vi "TenGbE_FPGA.vi"() -> ()   [LabVIEW 2017, in "My Network FPGA v1.lvlib"]
uses:
  Example SubVIs/My Network FPGA v1.lvlib
  <instrlib>/_niInstr/Streaming/v1/Common/Stream State.ctl
  <vilib>/Platform/TimedLoop/XDataNode/timing_clust.ctl
  <vilib>/Platform/TimedLoop/XDataNode/nitl_modes.ctl
  <vilib>/Platform/TimedLoop/XDataNode/wakeup.ctl
  <instrlib>/_niInstr/Network/Ethernet/MAC/CLIP/v1/Resources.ctl
  Example SubVIs/TX Controls.ctl
  <instrlib>/_niInstr/Network/Ethernet/MAC/CLIP/v1/niInstr Ethernet MAC - CLIP v1.lvclass
  C:/Program Files (x86)/National Instruments/LabVIEW 2017/instr.lib/_niInstr/Network/Ethernet/MAC/API/v1/FPGA/niInstr Ethernet MAC v1.lvclass
  <instrlib>/_niInstr/Network/API/v1/FPGA/Address Space/niInstr Network API FPGA Address Space v1.lvclass
  C:/Program Files (x86)/National Instruments/LabVIEW 2017/instr.lib/_niInstr/Instruction Framework/v1/FPGA/Interfaces/Address Space Collection/Address Space Collection.lvclass
  <instrlib>/_niInstr/FIFO Register Bus/v1/FPGA/niInstr FIFO Register Bus v1 FPGA.lvclass
  C:/Program Files (x86)/National Instruments/LabVIEW 2017/instr.lib/_niInstr/Instruction Framework/v1/FPGA/Interfaces/Instruction Producer/Instruction Producer.lvclass
  <vilib>/rvi/Emulation/niFpgaSctlEmulationGetInTimedLoop.vi
  <vilib>/rvi/Emulation/niFpgaEmulationReportErrorSimple.vi
  <vilib>/rvi/Emulation/niFpgaGetClockAttributes.vi
  <vilib>/rvi/Emulation/niFpgaCriticalErrorInLSC.vi
  <vilib>/rvi/Emulation/niFpgaProcessEmulError.vi
  <vilib>/rvi/eio/common/nirviEmuTemplateMethod_errors.vi
  <vilib>/Platform/TimedLoop/XDataNode/XDataNode.xnode
  <vilib>/eio/EIONode/EIONode.xnode
  <vilib>/Platform/TimedLoop/XDataNode/XDNodeRunTimeDep.lvlib
  <instrlib>/_niInstr/Instruction Framework/v1/FPGA/Top Level Bus/Register Configuration/Register Configuration.lvclass
  <instrlib>/_niInstr/Network/API/v1/FPGA/niInstr Network API FPGA v1.lvclass
  <instrlib>/_niInstr/Streaming/v1/Common/niInstr Streaming v1 Common.lvlib
panel:
  out "d_microblaze\\AXI_STR_RXD_1_tready":bool
  out "d_microblaze\\AXI_STR_RXD_tready":bool
  out "d_microblaze\\AXI_STR_TXD_1_tdata":fxp<+,32,32>
  out "d_microblaze\\AXI_STR_TXD_1_tlast":bool
  out "d_microblaze\\AXI_STR_TXD_1_tvalid":bool
  out "d_microblaze\\AXI_STR_TXD_tdata":fxp<+,32,32>
  out "d_microblaze\\AXI_STR_TXD_tlast":bool
  out "d_microblaze\\AXI_STR_TXD_tvalid":bool
  out "d_microblaze\\gpio1_out_tri_o":fxp<+,32,32>
  out "d_microblaze\\gpio2_out_tri_o":fxp<+,32,32>
  in  "Tab Control":T1(tab)
  in  "UDP Source Port 0":u16=43981
  in  "UDP Destination Port 0":u16=61185
  in  "preferred datagram size 0":u16=1472
  in  "Port 0 RX/TX":enum32{"RX", "TX"}(tab)
  in  "Port 0 RAW Mode":bool
  in  "Port 0 RX Clear Counts":bool
  out "Port 0 RX Good Frames Count":u32
  out "Port 0 RX Error Frames Count":u32
  out "Port 0 RX Received Columns Count":u32
  out "Port 0 RX Dropped Columns Count":u32
  out "Port 0 RX Data":u64 format="%.0x"
  in  "stream.num samples 0":u64
  in  "stream.request state 0":T2
  out "stream.metadata 0":u64
  out "stream.samples transferred 0":u64
  out "stream.state 0":T2
  in  "UDP Source Port 1":u16=43981
  in  "UDP Destination Port 1":u16=61185
  in  "preferred datagram size 1":u16=1472
  in  "Port 1 RX/TX":enum32{"RX", "TX"}(tab)
  in  "Port 1 RAW Mode":bool
  in  "Port 1 RX Clear Counts":bool
  out "Port 1 RX Dropped Columns Count":u32
  out "Port 1 RX Received Columns Count":u32
  out "Port 1 RX Error Frames Count":u32
  out "Port 1 RX Good Frames Count":u32
  out "Port 1 RX Data":u64 format="%.0x"
  in  "stream.request state 1":T2 caption="stream.request state 0"
  in  "stream.num samples 1":u64 caption="stream.num samples 0"
  out "stream.state 1":T2 caption="stream.state 0"
  out "stream.samples transferred 1":u64 caption="stream.samples transferred 0"
  out "stream.metadata 1":u64 caption="stream.metadata 0"
  in  "Use Pattern Gen":bool
  in  "max frame payload":u16=1472
  in  "minimum packet interval":u32=1
  out "mgtrefclks_locked":bool
  out "mgtrefclks_valid":bool
  out "posc_complete":bool
  out "aBlockLockPort0":bool
  out "aBlockLockPort1":bool
  out "sPort0_Power_Good":bool
  out "sPort1_Power_Good":bool
  out "signal_detect_Port0":bool
  out "signal_detect_Port1":bool
  in  "fifo reg bus ctrl 0":u32
  out "fifo reg bus status 0":u32
  out "fifo reg bus data 0":u64
  # "License Note\n\nThis example makes use of code under the LGPLv2 license in the Socketed CLIP to support 10 Gigabit Ethernet.  You may find the source and build instructions for this component in the CLIP directory."
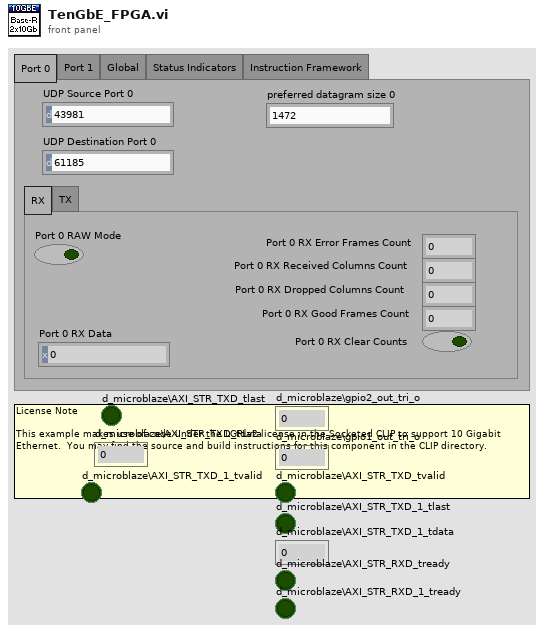
[diagram p1: front panel]
types:
  T1 = enum32{"Port 0", "Port 1", "Global", "Status Indicators", "Instruction Framework"}
  T2 = typedef "niInstr Streaming v1 Common.lvlib/Stream State.ctl" = enum8{"Idle", "Finite Transfer", "Continuous", "Done", "Error", "Not Ready", "Cancel"}
  T3 = typedef "niInstr Ethernet MAC - CLIP v1.lvclass/Resources.ctl" = cluster{"RX":cluster{"TData":refnum<k21>, "TValid":refnum<k21>, "TKeep":refnum<k21>, "TLast":refnum<k21>, "TUser":refnum<k21>}, "TX":cluster{"TData":refnum<k21>, "TValid":refnum<k21>, "TKeep":refnum<k21>, "TLast":refnum<k21>, "TReady":refnum<k21>}, "Pause resources":cluster{"cPauseValuePort":refnum<k21>, "cPauseReqPort":refnum<k21>}, "MAC Clock":refnum<k21>}
  T4 = typedef "XDNodeRunTimeDep.lvlib/timing_clust.ctl" = cluster{"Expected End [f-1]":u64, "Actual End [f-1]":u64, "Finished Late? [f-1]":bool, "Expected End [i-1]":u64, "Actual End [i-1]":u64, "Finished Late? [i-1]":bool, "Expected Start [i]":u64, "Actual Start [i]":u64, "Expected Start [f]":u64, "Actual Start [f]":u64, "Source Name":string, "Structure Name":string, "Period":i64, "Deadline":i64, "Offset":i64, "Start":i64, "Priority":i32, "Timeout":i32, "Mode":T5, "Wakeup Reason":T6, "Error":errorcluster, "Source Type":string, "Secondary Source Type":string, "Global End Time":u64, "Global Start Time":u64, "Frame Duration":u64, "Iteration Duration":u64, "Assigned CPU":i32, "I/O Scan Engine Mode":u32}
  T5 = typedef "XDNodeRunTimeDep.lvlib/nitl_modes.ctl" = enum32{"No Change", "Process missed periods, maintain original phase", "Discard missed periods, maintain original phase", "Process missed periods, ignore original phase", "Discard missed periods, ignore original phase"}
  T6 = typedef "XDNodeRunTimeDep.lvlib/wakeup.ctl" = enum32{"Normal", "Aborted", "Asynchronous wakeup", "Timing source error", "Timed loop error", "Timeout"}
  T7 = typedef "My Network FPGA v1.lvlib/TX Controls.ctl" = cluster{"UDP Source Port":u16, "UDP Destination Port":u16, "preferred datagram size":u16, "Use Pattern Gen":bool, "max frame payload":u16, "minimum packet interval":u32, "stream.num samples 0":u64, "stream.request state 0":T2}
  T8 = cluster{"Port RX Good Frames Count":u32, "Port RX Received Columns Count":u32, "Port RX Dropped Columns Count":u32, "Port RX Error Frames Count":u32, "Port RX Data":u64}
  T9 = typedef "My Network FPGA v1.lvlib/TX Indicators.ctl" = cluster{"stream.state 0":T2, "stream.metadata 0":u64, "stream.samples transferred 0":u64}
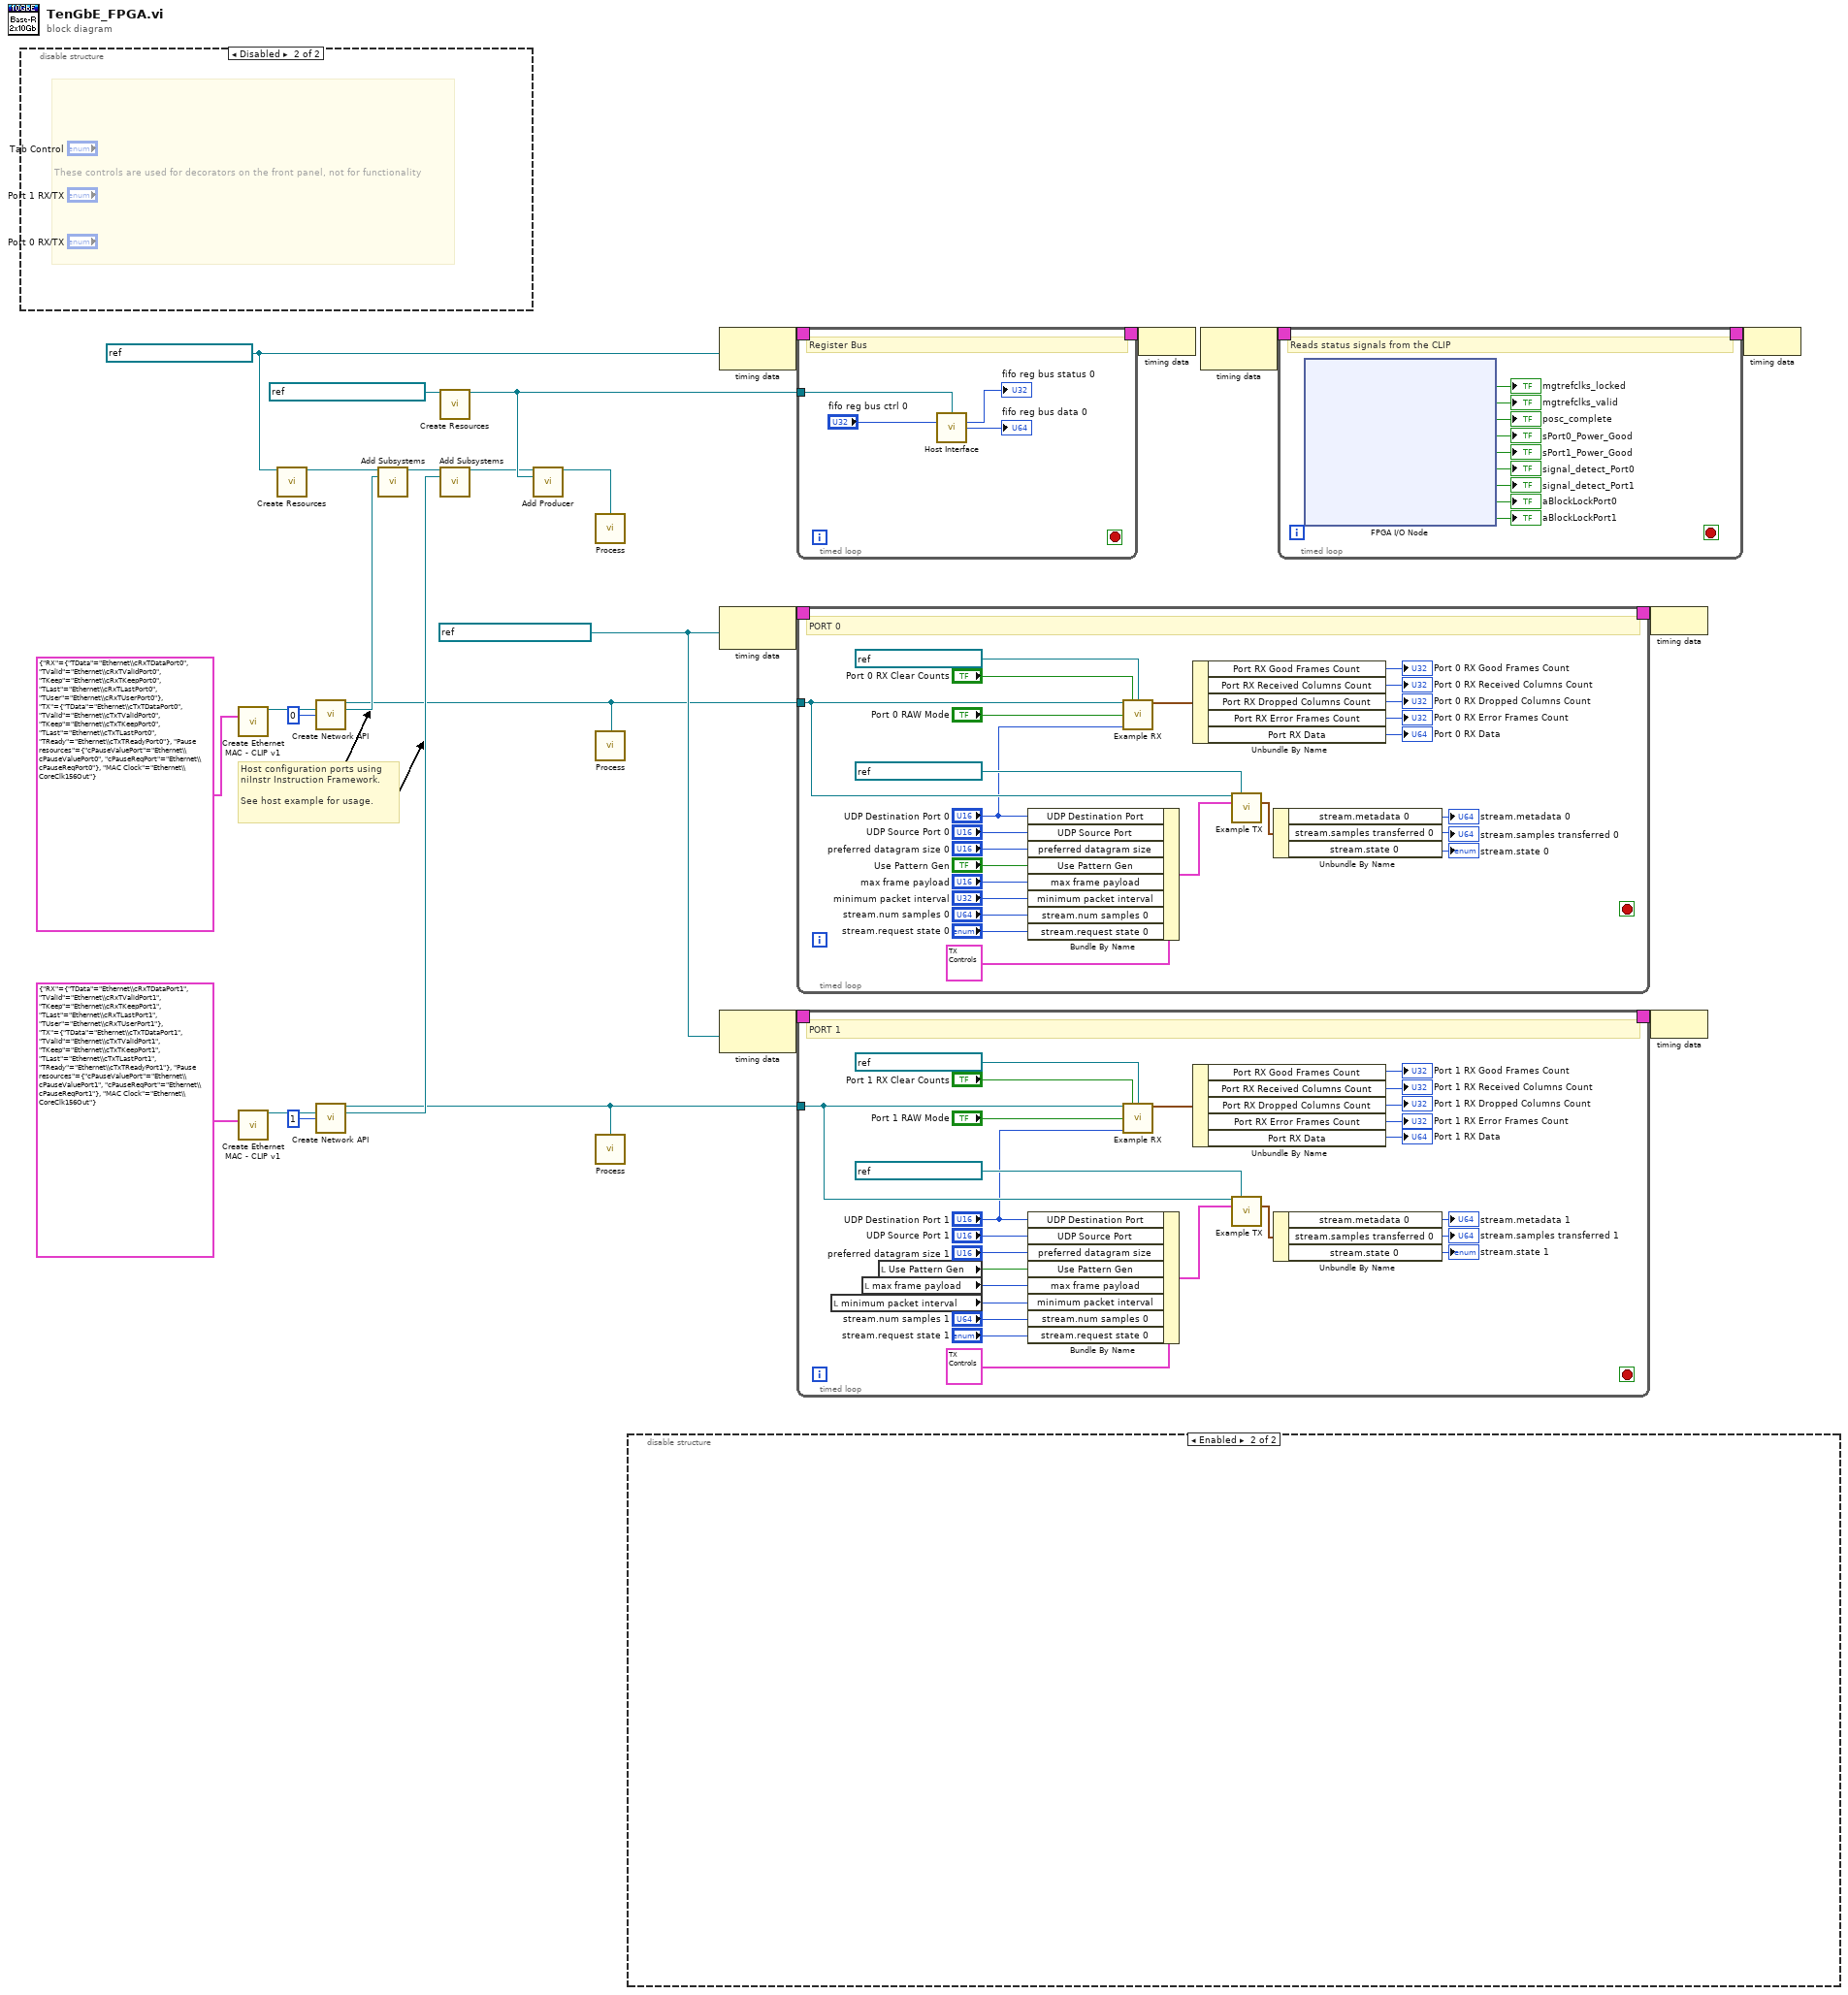
[diagram p0: block diagram]
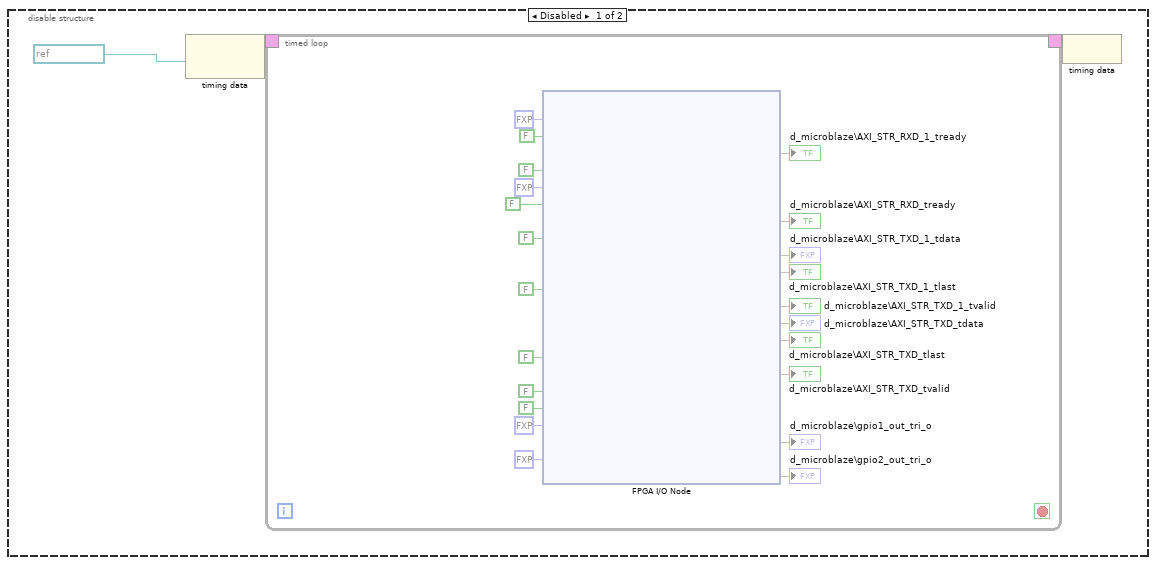
[diagram p2: hidden frame]
diagram:
  w5 = refnum<k21> "Ethernet\\CoreClk156Out" ("Source Name")
  w21 = refnum<k21> "40 MHz Onboard Clock" ("Source Name")
  # "Host configuration ports using\nniInstr Instruction Framework.\n\nSee host example for usage."
  n1 = disable-structure shown="Disabled" {
    frame Enabled {
    }
    frame Disabled {
      # "These controls are used for decorators on the front panel, not for functionality"
    }
  }
  n2 = call <instrlib>:"Create Ethernet MAC - CLIP v1.vi"("Ethernet AXI4-S Resources"=T3 {"RX"={"TData"="Ethernet\\cRxTDataPort0", "TValid"="Ethernet\\cRxTValidPort0", "TKeep"="Ethernet\\cRxTKeepPort0", "TLast"="Ethernet\\cRxTLastPort0", "TUser"="Ethernet\\cRxTUserPort0"}, "TX"={"TData"="Ethernet\\cTxTDataPort0", "TValid"="Ethernet\\cTxTValidPort0", "TKeep"="Ethernet\\cTxTKeepPort0", "TLast"="Ethernet\\cTxTLastPort0", "TReady"="Ethernet\\cTxTReadyPort0"}, "Pause resources"={"cPauseValuePort"="Ethernet\\cPauseValuePort0", "cPauseReqPort"="Ethernet\\cPauseReqPort0"}, "MAC Clock"="Ethernet\\CoreClk156Out"}) -> ("niInstr Ethernet MAC - CLIP v1.lvclass out"=w16:refnum<class "niInstr Ethernet MAC - CLIP v1.lvclass">)  [unwired: 14 in]
  n3 = call <instrlib>:"Create Ethernet MAC - CLIP v1.vi"("Ethernet AXI4-S Resources"=T3 {"RX"={"TData"="Ethernet\\cRxTDataPort1", "TValid"="Ethernet\\cRxTValidPort1", "TKeep"="Ethernet\\cRxTKeepPort1", "TLast"="Ethernet\\cRxTLastPort1", "TUser"="Ethernet\\cRxTUserPort1"}, "TX"={"TData"="Ethernet\\cTxTDataPort1", "TValid"="Ethernet\\cTxTValidPort1", "TKeep"="Ethernet\\cTxTKeepPort1", "TLast"="Ethernet\\cTxTLastPort1", "TReady"="Ethernet\\cTxTReadyPort1"}, "Pause resources"={"cPauseValuePort"="Ethernet\\cPauseValuePort1", "cPauseReqPort"="Ethernet\\cPauseReqPort1"}, "MAC Clock"="Ethernet\\CoreClk156Out"}) -> ("niInstr Ethernet MAC - CLIP v1.lvclass out"=w13:refnum<class "niInstr Ethernet MAC - CLIP v1.lvclass">)  [unwired: 14 in]
  n4 = call <instrlib>:"Create Resources.vi"("register clock"=w21) -> ("register configuration"=w15:refnum<class "Register Configuration.lvclass">)  [unwired: 14 in]
  n5 = call <instrlib>:"Create Network API.vi"("niInstr Ethernet MAC v1.lvclass"=w16, "instance"=u8 0 ("Instance")) -> ("niInstr Network API FPGA v1.lvclass"=w1:refnum<class "niInstr Network API FPGA v1.lvclass">, "Address Space Collection"=w14:refnum<class "niInstr Network API FPGA Address Space v1.lvclass">)  [unwired: 12 in]
  n6 = call <instrlib>:"Create Network API.vi"("niInstr Ethernet MAC v1.lvclass"=w13, "instance"=u8 1 ("Instance")) -> ("niInstr Network API FPGA v1.lvclass"=w4:refnum<class "niInstr Network API FPGA v1.lvclass">, "Address Space Collection"=w11:refnum<class "niInstr Network API FPGA Address Space v1.lvclass">)  [unwired: 12 in]
  n7 = call <instrlib>:"Add Subsystems.vi"("register configuration in"=w15, "subsystems"=w14) -> ("register configuration out"=w12:refnum<class "Register Configuration.lvclass">)  [unwired: 13 in]
  n8 = call <instrlib>:"Create Resources.vi"("instruction fifo"=refnum<k21> "reg.host instruction fifo 0" ("FIFO")) -> ("fifo register bus"=w20:refnum<class "niInstr FIFO Register Bus v1 FPGA.lvclass">)  [unwired: 14 in]
  n9 = call <instrlib>:"Add Subsystems.vi"("register configuration in"=w12, "subsystems"=w11) -> ("register configuration out"=w8:refnum<class "Register Configuration.lvclass">)  [unwired: 13 in]
  n10 = call <instrlib>:"Add Producer.vi"("register configuration in"=w8, "instruction producer"=w20) -> ("register configuration out"=w19:refnum<class "Register Configuration.lvclass">)  [unwired: 13 in]
  n11 = call <instrlib>:"Process.vi"("register configuration"=w19) -> ()  [unwired: 15 in]
  n12 = call <instrlib>:"Process.vi"("niInstr Network API FPGA v1.lvclass"=w1) -> ()  [unwired: 15 in]
  n13 = call <instrlib>:"Process.vi"("niInstr Network API FPGA v1.lvclass"=w4) -> ()  [unwired: 15 in]
  n14 = disable-structure shown="Enabled" {
    frame Disabled {
      n15 = node-c288(refnum<k21> "100MHz" ("Source Name")) -> (w29:T4)
      n16 = timed-loop {
        timing: w29 -> [_]
        timing-out: [_] -> w28
        stop <- _ stop-if-true
        n17 = xnode "FPGA I/O Node"("d_microblaze\\AXI_STR_RXD_1_tdata"=fxp<+,32,32> 0.0 ("d_microblaze\\AXI_STR_RXD_1_tdata"), "d_microblaze\\AXI_STR_RXD_1_tlast"=FALSE ("d_microblaze\\AXI_STR_RXD_1_tlast"), "d_microblaze\\AXI_STR_RXD_1_tvalid"=FALSE ("d_microblaze\\AXI_STR_RXD_1_tvalid"), "d_microblaze\\AXI_STR_RXD_tdata"=fxp<+,32,32> 0.0 ("d_microblaze\\AXI_STR_RXD_tdata"), "d_microblaze\\AXI_STR_RXD_tlast"=FALSE ("d_microblaze\\AXI_STR_RXD_tlast"), "d_microblaze\\AXI_STR_RXD_tvalid"=FALSE ("d_microblaze\\AXI_STR_RXD_tvalid"), "d_microblaze\\AXI_STR_TXD_1_tready"=FALSE ("d_microblaze\\AXI_STR_TXD_1_tready"), "d_microblaze\\AXI_STR_TXD_tready"=FALSE ("d_microblaze\\AXI_STR_TXD_tready"), "d_microblaze\\Int_0"=FALSE ("d_microblaze\\Int_0"), "d_microblaze\\Int_1"=FALSE ("d_microblaze\\Int_1"), "d_microblaze\\gpio1_in_tri_i"=fxp<+,32,32> 0.0 ("d_microblaze\\gpio1_in_tri_i"), "d_microblaze\\gpio2_in_tri_i"=fxp<+,32,32> 0.0 ("d_microblaze\\gpio2_in_tri_i")) -> ("d_microblaze\\AXI_STR_RXD_1_tready"=→"d_microblaze\\AXI_STR_RXD_1_tready", "d_microblaze\\AXI_STR_RXD_tready"=→"d_microblaze\\AXI_STR_RXD_tready", "d_microblaze\\AXI_STR_TXD_1_tdata"=→"d_microblaze\\AXI_STR_TXD_1_tdata", "d_microblaze\\AXI_STR_TXD_1_tlast"=→"d_microblaze\\AXI_STR_TXD_1_tlast", "d_microblaze\\AXI_STR_TXD_1_tvalid"=→"d_microblaze\\AXI_STR_TXD_1_tvalid", "d_microblaze\\AXI_STR_TXD_tdata"=→"d_microblaze\\AXI_STR_TXD_tdata", "d_microblaze\\AXI_STR_TXD_tlast"=→"d_microblaze\\AXI_STR_TXD_tlast", "d_microblaze\\AXI_STR_TXD_tvalid"=→"d_microblaze\\AXI_STR_TXD_tvalid", "d_microblaze\\gpio1_out_tri_o"=→"d_microblaze\\gpio1_out_tri_o", "d_microblaze\\gpio2_out_tri_o"=→"d_microblaze\\gpio2_out_tri_o")  [unwired: 22 in, 22 out]
      }
      n18 = node-c288(w28) -> ()
    }
    frame Enabled {
    }
  }
  n19 = node-c288(w21) -> (w24:T4)
  n20 = node-c288(w5) -> (w18:T4)
  n21 = node-c288(w5) -> (w7:T4)
  n22 = timed-loop {
    timing: w24 -> [_]
    timing-out: [_] -> w23
    tunnel: w20 -> [w61]
    stop <- _ stop-if-true
    # "Register Bus"
    n23 = call <instrlib>:"Host Interface.vi"("fifo register bus"=w61, "fifo reg bus ctrl 0"="fifo reg bus ctrl 0") -> ("fifo reg bus status 0"=→"fifo reg bus status 0":u32, "fifo reg bus data 0"=→"fifo reg bus data 0":u64)  [unwired: 12 in]
  }
  n24 = timed-loop {
    timing: w18 -> [_]
    timing-out: [_] -> w17
    tunnel: w1 -> [w80]
    stop <- _ stop-if-true
    # "PORT 0"
    n25 = Bundle By Name(cluster=T7 {"UDP Source Port"=43981, "UDP Destination Port"=61185, "preferred datagram size"=1400, "Use Pattern Gen"=FALSE, "max frame payload"=1472, "minimum packet interval"=1, "stream.num samples 0"=0, "stream.request state 0"=enum."Idle"} ("Controls"), "UDP Destination Port"="UDP Destination Port 0", "UDP Source Port"="UDP Source Port 0", "preferred datagram size"="preferred datagram size 0", "Use Pattern Gen"="Use Pattern Gen", "max frame payload"="max frame payload", "minimum packet interval"="minimum packet interval", "stream.num samples 0"="stream.num samples 0", "stream.request state 0"="stream.request state 0") -> (w78:T7)
    n26 = call "Example RX.vi"("niInstr Network API FPGA v1.lvclass"=w80, "Port RX Clear Counts"="Port 0 RX Clear Counts", "Host RX FIFO"=refnum<k21> "Port 0 Host RX FIFO", "RAW Mode"="Port 0 RAW Mode", "Dest Port"="UDP Destination Port 0") -> ("debug data"=w87:T8)  [unwired: 10 in]
    n27 = Unbundle By Name(w87) -> ("Port RX Good Frames Count"=→"Port 0 RX Good Frames Count":u32, "Port RX Received Columns Count"=→"Port 0 RX Received Columns Count":u32, "Port RX Dropped Columns Count"=→"Port 0 RX Dropped Columns Count":u32, "Port RX Error Frames Count"=→"Port 0 RX Error Frames Count":u32, "Port RX Data"=→"Port 0 RX Data":u64)
    n28 = call "Example TX.vi"("Network API"=w80, "FIFO In"=refnum<k21> "Port 0 Host TX FIFO", "Controls"=w78) -> ("Indicators"=w70:T9)  [unwired: 12 in]
    n29 = Unbundle By Name(w70) -> ("stream.metadata 0"=→"stream.metadata 0":u64, "stream.samples transferred 0"=→"stream.samples transferred 0":u64, "stream.state 0"=→"stream.state 0":T2)
  }
  n30 = timed-loop {
    timing: w7 -> [_]
    timing-out: [_] -> w6
    tunnel: w4 -> [w103]
    stop <- _ stop-if-true
    # "PORT 1"
    n31 = local read "minimum packet interval"() -> (w98:u32)
    n32 = local read "max frame payload"() -> (w99:u16)
    n33 = local read "Use Pattern Gen"() -> (w100:bool)
    n34 = Bundle By Name(cluster=T7 {"UDP Source Port"=43981, "UDP Destination Port"=61185, "preferred datagram size"=1400, "Use Pattern Gen"=FALSE, "max frame payload"=1472, "minimum packet interval"=1, "stream.num samples 0"=0, "stream.request state 0"=enum."Idle"} ("Controls"), "UDP Destination Port"="UDP Destination Port 1", "UDP Source Port"="UDP Source Port 1", "preferred datagram size"="preferred datagram size 1", "Use Pattern Gen"=w100, "max frame payload"=w99, "minimum packet interval"=w98, "stream.num samples 0"="stream.num samples 1", "stream.request state 0"="stream.request state 1") -> (w105:T7)
    n35 = call "Example RX.vi"("niInstr Network API FPGA v1.lvclass"=w103, "Port RX Clear Counts"="Port 1 RX Clear Counts", "Host RX FIFO"=refnum<k21> "Port 1 Host RX FIFO", "RAW Mode"="Port 1 RAW Mode", "Dest Port"="UDP Destination Port 1") -> ("debug data"=w115:T8)  [unwired: 10 in]
    n36 = Unbundle By Name(w115) -> ("Port RX Good Frames Count"=→"Port 1 RX Good Frames Count":u32, "Port RX Received Columns Count"=→"Port 1 RX Received Columns Count":u32, "Port RX Dropped Columns Count"=→"Port 1 RX Dropped Columns Count":u32, "Port RX Error Frames Count"=→"Port 1 RX Error Frames Count":u32, "Port RX Data"=→"Port 1 RX Data":u64)
    n37 = call "Example TX.vi"("Network API"=w103, "FIFO In"=refnum<k21> "Port 1 Host TX FIFO", "Controls"=w105) -> ("Indicators"=w106:T9)  [unwired: 12 in]
    n38 = Unbundle By Name(w106) -> ("stream.metadata 0"=→"stream.metadata 1":u64, "stream.samples transferred 0"=→"stream.samples transferred 1":u64, "stream.state 0"=→"stream.state 1":T2)
  }
  n39 = node-c288(w23) -> ()
  n40 = node-c288() -> (w26:T4)  [unwired: 1 in]
  n41 = timed-loop {
    timing: w26 -> [_]
    timing-out: [_] -> w25
    stop <- _ stop-if-true
    # "Reads status signals from the CLIP"
    n42 = xnode "FPGA I/O Node"() -> ("Ethernet\\MgtRefClks_Locked"=→"mgtrefclks_locked":bool, "Ethernet\\MgtRefClks_Valid"=→"mgtrefclks_valid":bool, "Ethernet\\POSC_Complete"=→"posc_complete":bool, "Ethernet\\sPort0_Power_Good"=→"sPort0_Power_Good":bool, "Ethernet\\sPort1_Power_Good"=→"sPort1_Power_Good":bool, "Ethernet\\signal_detect_Port0"=→"signal_detect_Port0":bool, "Ethernet\\signal_detect_Port1"=→"signal_detect_Port1":bool, "Ethernet\\aBlockLockPort0"=→"aBlockLockPort0":bool, "Ethernet\\aBlockLockPort1"=→"aBlockLockPort1":bool)  [unwired: 9 in, 9 out]
  }
  n43 = node-c288(w17) -> ()
  n44 = node-c288(w6) -> ()
  n45 = node-c288(w25) -> ()
